vi "Sequencer Main.vi"() -> ()   [LabVIEW 2018] (continued)
                            n2810 = Replace Array Subset(array=w5930, new element=w5928, index=10) -> (w5931:errorcluster[])
                            n2811 = global write "Global Variable.vi" "Array Errors"(w5931) -> ()
                          }
                          n2812 = case shown="True" w5908 {
                            tunnel: [enum16{"Idle", "PASS", "FALSE"}."FALSE" ("Step Test Result") enum16{"Idle", "PASS", "FALSE"}."PASS" ("Step Test Result")] -> w5907
                            tunnel: ["FLASH FALSE" "FLASH OK"] -> w5904
                            frame False {
                              # "Step TEST Result"
                            }
                            frame True {
                              # "Step TEST Result"
                            }
                          }
                          n2813 = in-place {
                            in-place-border: w5906 -> [w5919]
                            in-place-border: w5905 -> [w5918]
                            in-place-border: w5904 -> [w5917]
                            n2814 = call "Log Add Msg.vi"("Result"=w5917, "Communication"=w5918, "Description"=w5919) -> ("Out Msg"=w5920:string)
                            n2815 = property on="LogMsg" class="Str"("Text.Scroll Position"=inf) -> ()  [unwired: 2 in, 2 out]
                            n2816 = invoke on="LogMsg" class="Str" method="Append String"("string"=w5920) -> ()  [unwired: 3 in, 4 out]
                          }
                        }
                        frame 1000 {
                          # "Power Supply OFF, Reset DIO"
                          # "Step TEST Result"
                          # "RESET POWER SUPPLY & RESET GPIO"
                          n2817 = Unbundle By Name(w5941) -> ("Step Description"=w5940:string)
                          n2818 = Concatenate Strings(w5940, "  " ("string"), "<END OF SEQUENCER>" ("string")) -> (w5942:string)
                          n2819 = local write "Message"(w5942) -> ()
                          n2820 = property on="Tab Control Msg" class="TabCtl (strict)"("Value"=T21."Msg" ("Tab Control Msg")) -> (error out=w5935:errorcluster)  [unwired: 2 in, 1 out]
                          n2821 = flat-sequence {
                            tunnel: w5935 -> [_]
                            tunnel: w5934 -> [w5960]
                            tunnel: w5933 -> [w5959]
                            frame #0 {
                              w5945 = FALSE ("Enable Output")
                              w5943 = 0.1 ("Current")
                              w5944 = 0.0 ("Voltage")
                              n2822 = global read "Global Variable.vi" "VISA Resource Name BK-9202"() -> (w5954:string)
                              n2823 = call "bk9201 Set.vi"("Enable Output"=w5945, "Current"=w5943, "Voltage"=w5944, "VISA resource name"=w5954) -> ("error out"=w5950:errorcluster)  [unwired: 7 in]
                              n2824 = local read "PowSupply - SET"() -> (w5947:T7)
                              n2825 = local read "Switch Relay Modules"() -> (w5949:T5)
                              n2826 = Bundle By Name(cluster=w5949, "Main Power Supplay ON/OFF"=w5945) -> (w5948:T5)
                              n2827 = global read "Global Variable.vi" "Array Errors"() -> (w5952:errorcluster[])
                              n2828 = Bundle By Name(cluster=w5947, "ON/OFF"=w5945, "Volt (V)"=w5944, "Current Limit (A)"=w5943) -> (w5946:T7)
                              n2829 = global write "Global Variable.vi" "PowSupply ON/OFF"(w5945) -> ()
                              n2830 = Replace Array Subset(array=w5952, new element=w5950, index=2) -> (w5953:errorcluster[])
                              n2831 = local write "Switch Relay Modules"(w5948) -> ()
                              n2832 = local write "PowSupply - SET"(w5946) -> ()
                              n2833 = global write "Global Variable.vi" "Array Errors"(w5953) -> ()
                            }
                            frame #1 {
                              n2834 = call <vilib>:"Acquire Semaphore.vi"("error in (no error)"=w5960, "semaphore"=w5959) -> ("error out"=w5958:errorcluster, "semaphore out"=w5956:T13)  [unwired: 3 in, 1 out]
                              n2835 = case shown="No Error" w5958 {
                                selector: w5958 -> [w5962 w5981]
                                tunnel: [w5962 w5981] -> w5955
                                tunnel: [w5961 w5980] -> w5957
                                tunnel: w5956 -> [w5961 w5980]
                                frame No Error {
                                n2836 = disable-structure shown="Disabled" {
                                frame Disabled {
                                n2837 = local read "Switch Relay Modules"() -> (w5970:T5)
                                n2838 = Number To Boolean Array(number=u16 0) -> (Boolean array=w5972:bool[])
                                n2839 = Bundle By Name(cluster=w5970, "SW 0"=w5972, "SW 1"=w5972, "SW 2"=w5972, "SW 3"=w5972, "SW 4"=w5972, "SW 5"=w5972, "SW 6"=w5972) -> (w5971:T5)
                                n2840 = local write "Switch Relay Modules"(w5971) -> ()
                                }
                                frame Enabled {
                                }
                                }
                                n2841 = global read "Global Variable.vi" "FTDI SPI Handle"() -> (w5965:u32)
                                n2842 = for {
                                N: 7 -> [_]
                                tunnel: w5965 -> [w5978]
                                tunnel: [w5979] -> w5968
                                i -> [w5973]
                                w5975 = u8 0  # nCS
                                w5974 = u16 0  # Channel Decimal
                                w5976 = FALSE  # Use Extra
                                n2843 = call "FTDI SPI GPIO Set.vi"("nCS"=w5975, "Mode"=T23."Set Decimal", "Use Extra"=w5976, "Channel Decimal"=w5974, "Addr"=w5973, "Handler In"=w5978) -> ("error out"=w5979:errorcluster)  [unwired: 2 in, 3 out]
                                }
                                n2844 = global read "Global Variable.vi" "Array Errors"() -> (w5966:errorcluster[])
                                n2845 = Replace Array Subset(array=w5966, new element=w5968, index=10) -> (w5967:errorcluster[])
                                n2846 = global write "Global Variable.vi" "Array Errors"(w5967) -> ()
                                }
                                frame Error {
                                }
                              }
                              n2847 = call <vilib>:"Release Semaphore.vi"("error in (no error)"=w5955, "semaphore"=w5957) -> ()  [unwired: 4 in, 2 out]
                            }
                            frame #2 {
                              w5982 = "!END OF TEST\nReset ALL"
                              n2848 = local write "Message"(w5982) -> ()
                              n2849 = property on="Msg Str" class="Str"("Value"=w5982) -> ()  [unwired: 2 in, 2 out]
                            }
                          }
                        }
                      }
                    }
                  }
                }
                frame #1 {
                  # "Step Result Msg"
                  # "Report"
                  # "Step TEST Result"
                  # "Run/Skip"
                  # "Step Type"
                  # "PASS/FALSE"
                  n2850 = Unbundle By Name(w5997) -> ("Run/Skip"=w5993:bool, "Step Type"=w5996:u16, "Report"=w5985:bool)
                  n2851 = flat-sequence {
                    tunnel: w5990 -> [w6002]
                    tunnel: w5983 -> [w6003]
                    tunnel: [w6005] -> w5995
                    tunnel: [w6004] -> w5994
                    tunnel: w5992 -> [w6000]
                    tunnel: [w6001] -> w5988
                    tunnel: w5995 -> [w6047]
                    tunnel: w5994 -> [w6048]
                    tunnel: w5983 -> [w6053]
                    tunnel: w5993 -> [w6049]
                    tunnel: w5991 -> [w6052]
                    tunnel: [w6051] -> w5984
                    tunnel: [w6050] -> w5989
                    tunnel: w5988 -> [w6050]
                    tunnel: w5983 -> [w6085]
                    tunnel: w5990 -> [w6084]
                    tunnel: w5989 -> [w6080]
                    tunnel: [w6079] -> w5986
                    tunnel: [w6114] -> w5987
                    tunnel: w5986 -> [w6114]
                    frame #0 {
                      # "BREACK ON FIRST Err"
                      n2852 = flat-sequence {
                        tunnel: w6000 -> [w6007]
                        tunnel: w6002 -> [w6008]
                        tunnel: w6003 -> [w6006]
                        tunnel: [w6008] -> w5999
                        tunnel: [w6007] -> w5998
                        tunnel: [w6019] -> w6005
                        tunnel: [w6018] -> w6004
                        tunnel: [w6016] -> w6001
                        tunnel: w5999 -> [w6017]
                        tunnel: w5998 -> [w6015]
                        frame #0 {
                          n2853 = case shown="\"FALSE\"" w6006 {
                            frame "Idle", Default {
                            }
                            frame "FALSE" {
                              n2854 = in-place {
                                in-place-border: [w6010] -> w6009
                                n2855 = global read "Global Variable.vi" "Retest Cnt"() -> (w6011:i16)
                                n2856 = Equal?(x=w6011, y=i16 0) -> (x = y?=w6010:bool)
                              }
                              n2857 = case shown="True" w6009 {
                                frame False {
                                }
                                frame True {
                                n2858 = global read "Global Variable.vi" "Gen Err Cnt"() -> (w6014:u16)
                                n2859 = Increment(x=w6014) -> (x+1=w6013:u16)
                                n2860 = global write "Global Variable.vi" "Gen Err Cnt"(w6013) -> ()
                                }
                              }
                            }
                          }
                        }
                        frame #1 {
                          # "GoTo  the last Sekuencer STEP (test Id=1000)"
                          n2861 = in-place {
                            in-place-border: [w6031] -> w6016
                            in-place-border: [w6029] -> w6019
                            in-place-border: [w6028] -> w6018
                            in-place-border: w6017 -> [w6027]
                            in-place-border: w6015 -> [w6026]
                            # "And"
                            # "Break On 3xFirst Err"
                            n2862 = global read "Global Variable.vi" "Gen Err Cnt"() -> (w6025:u16)
                            n2863 = Greater Or Equal?(x=w6025, y=u16 3) -> (x >= y?=w6021:bool)
                            n2864 = And(x=w6021, y="Break On First Err") -> (x .and. y?=w6022:bool)
                            n2865 = case shown="True" w6022 {
                              tunnel: [FALSE TRUE] -> w6023
                              frame False {
                              }
                              frame True {
                                n2866 = global write "Global Variable.vi" "Test Gen Status"(FALSE ("Test Gen Status")) -> ()
                              }
                            }
                            n2867 = And(x=w6023, y="Break On First Err") -> (x .and. y?=w6030:bool)
                            n2868 = case shown="True" w6030 {
                              tunnel: w6027 -> [_ w6045]
                              tunnel: w6026 -> [w6037 w6046]
                              tunnel: [w6037 w6042] -> w6031
                              tunnel: [FALSE TRUE] -> w6029
                              tunnel: [0 w6038] -> w6028
                              frame False {
                              }
                              frame True {
                                n2869 = global read "Sequencer Array.vi" "SEQUENCER Array"() -> (w6044:T16[])
                                n2870 = Flush Queue(queue=w6045, error in (no error)=w6046) -> (queue out=w6043:refnum<queue>, error out=w6041:errorcluster)  [unwired: 1 out]
                                n2871 = Array Size(array=w6044) -> (size(s)=w6040:i32)
                                n2872 = Decrement(x=w6040) -> (x-1=w6038:i32)
                                n2873 = property on="Test Sequencer" class="MCListbox (strict)"("Value"=w6038) -> ()  [unwired: 2 in, 2 out]
                                n2874 = Enqueue Element(queue=w6043, element=w6038, error in (no error)=w6041) -> (error out=w6042:errorcluster)  [unwired: 1 in, 2 out]
                              }
                            }
                          }
                        }
                      }
                    }
                    frame #1 {
                      # "Step TEST Result"
                      # "Run/Skip & Retest-ON"
                      # "Fill-Up (PASS/FALSE)Test Sequenser Table"
                      n2875 = case shown="True" w6047 {
                        tunnel: w6048 -> [_ w6056]
                        frame False {
                        }
                        frame True {
                          # "Break on first Err jump"
                          n2876 = Add(x=w6056, y=-5) -> (x+y=w6055:i32)
                          n2877 = Bundle By Name(cluster=T14 {"Row"=0, "Column"=0} ("Top Left Visible Cell"), "Row"=w6055, "Column"=u32 0) -> (w6059:T14)
                          n2878 = property on="Test Sequencer" class="MCListbox (strict)"("TopLeft"=w6059) -> ()  [unwired: 2 in, 2 out]
                        }
                      }
                      n2879 = case shown="True" w6049 {
                        tunnel: w6053 -> [_ w6068]
                        tunnel: [u32 16448250 w6064] -> w6051
                        tunnel: w6052 -> [_ w6061]
                        frame False {
                        }
                        frame True {
                          w6069 = 5 ("disabled index (col)")
                          # "Step Result Msg"
                          # "A-1"
                          n2880 = case shown="\"FALSE\"" w6068 {
                            tunnel: [u32 16448250 u32 46115 u32 16711680] -> w6064
                            tunnel: ["Idle" "PASS" "FALSE"] -> w6067
                            frame "Idle", Default {
                            }
                            frame "PASS" {
                            }
                            frame "FALSE" {
                            }
                          }
                          n2881 = global read "Global Variable.vi" "Current Step Nmb"() -> (w6063:u32)
                          n2882 = property on="Test Squencer Edit" class="MCListbox (strict)"() -> ("ItemNames"=w6065:string[][])  [unwired: 2 in, 2 out]
                          n2883 = Bundle By Name(cluster=T15 {"Row"=0, "Column"=0} ("Active Cell:Active Cell"), "Row"=w6063, "Column"=w6069) -> (w6070:T15)
                          n2884 = Replace Array Subset(array=w6065, new element #1=w6067, index (row) #1=w6063, index (col) #1=w6069, new element #2=w6061, index (row) #2=w6063, index (col) #2=3 ("disabled index (col)")) -> (w6066:string[][])
                          n2885 = property on="Test Squencer Edit" class="MCListbox (strict)"("ItemNames"=w6066, "ActiveCell"=w6070, "CellFontColor"=w6064) -> ()  [unwired: 2 in, 2 out]
                        }
                      }
                    }
                    frame #2 {
                      # "Step TEST Result"
                      n2886 = global read "Global Variable.vi" "Retest Cnt"() -> (w6078:i16)
                      n2887 = global read "Global Variable.vi" "Retest ON"() -> (w6082:bool)
                      n2888 = Greater Than 0?(x=w6078) -> (x > 0?=w6081:bool)
                      n2889 = And(x=w6082, y=w6081) -> (x .and. y?=w6083:bool)
                      n2890 = case shown="True" w6083 {
                        tunnel: w6085 -> [_ w6090]
                        tunnel: w6084 -> [_ w6089]
                        tunnel: w6080 -> [w6086 w6088]
                        tunnel: [w6086 w6087] -> w6079
                        frame False {
                        }
                        frame True {
                          n2891 = case shown="\"FALSE\"" w6090 {
                            tunnel: [w6091 w6094 w6112] -> w6087
                            tunnel: w6089 -> [_ w6093 _]
                            tunnel: w6088 -> [w6091 w6092 w6112]
                            frame "Idle", Default {
                            }
                            frame "FALSE" {
                              n2892 = in-place {
                                in-place-border: w6093 -> [w6102]
                                in-place-border: w6092 -> [w6101]
                                in-place-border: [w6096] -> w6094
                                # "RETEST"
                                n2893 = global read "Global Variable.vi" "Retest Step Nmb"() -> (w6095:u32)
                                n2894 = global read "Global Variable.vi" "Steps Nmb"() -> (w6098:u32)
                                n2895 = disable-structure shown="Disabled" {
                                disable-tunnel: w6095 -> [w6103 _]
                                frame Disabled {
                                n2896 = Bundle By Name(cluster=T14 {"Row"=0, "Column"=0} ("Top Left Visible Cell"), "Row"=w6103) -> (w6104:T14)
                                n2897 = property on="Test Sequencer" class="MCListbox (strict)"("TopLeft"=w6104) -> ()  [unwired: 2 in, 2 out]
                                }
                                frame Enabled {
                                }
                                }
                                n2898 = Flush Queue(queue=w6102, error in (no error)=w6101) -> (queue out=w6099:refnum<queue>, error out=w6100:errorcluster)  [unwired: 1 out]
                                n2899 = property on="Test Sequencer" class="MCListbox (strict)"("Value"=w6095) -> ()  [unwired: 2 in, 2 out]
                                n2900 = Subtract(x=w6098, y=w6095) -> (x-y=w6097:u32)
                                n2901 = for {
                                N: w6097 -> [_]
                                tunnel: w6100 -> [w6111]
                                tunnel: w6099 -> [w6110]
                                tunnel: w6095 -> [w6107]
                                tunnel: [w6106] -> w6096
                                i -> [w6109]
                                n2902 = Add(x=w6107, y=w6109) -> (x+y=w6108:u32)
                                n2903 = Enqueue Element(queue=w6110, element=w6108, error in (no error)=w6111) -> (error out=w6106:errorcluster)  [unwired: 1 in, 2 out]
                                }
                              }
                            }
                            frame "PASS" {
                              n2904 = global write "Global Variable.vi" "Retest Cnt"(i16 0 ("Retest Cnt")) -> ()
                            }
                          }
                        }
                      }
                    }
                    frame #3 {
                      n2905 = in-place {
                        n2906 = global read "Global Variable.vi" "Retest Nmb"() -> (w6115:i16)
                        n2907 = global read "Global Variable.vi" "Retest Cnt"() -> (w6117:i16)
                        n2908 = Subtract(x=w6115, y=w6117) -> (x-y=w6116:i16)
                        n2909 = Number To Decimal String(number=w6116) -> (decimal integer string=w6119:string)  [unwired: 1 in]
                        n2910 = Greater Than 0?(x=w6117) -> (x > 0?=w6120:bool)
                        "RETEST" <- w6120
                        n2911 = global write "Global Variable.vi" "Retest ON"(FALSE ("Retest Start")) -> ()
                        n2912 = case shown="False" w6120 {
                          tunnel: w6119 -> [w6121 w6122]
                          frame False {
                            n2913 = property on="RETEST" class="Bool (strict)"("BoolText.Text"=w6121) -> ()  [unwired: 2 in, 2 out]
                          }
                          frame True {
                            n2914 = property on="RETEST" class="Bool (strict)"("BoolText.Text"=w6122) -> ()  [unwired: 2 in, 2 out]
                          }
                        }
                      }
                    }
                  }
                }
                frame #2 {
                  # "Report"
                  # "Run / Skip"
                  # "A-1"
                  # "REPORT GENERATION"
                  n2915 = global read "Global Variable.vi" "Retest Cnt"() -> (w6127:i16)
                  n2916 = Equal To 0?(x=w6127) -> (x = 0?=w6125:bool)
                  n2917 = in-place {
                    in-place-border: w6129 -> [w6132]
                    # "Error Store"
                    n2918 = global read "Global Variable.vi" "Array Errors"() -> (w6134:errorcluster[])
                    n2919 = Replace Array Subset(array=w6134, new element=w6132, index=7) -> (w6135:errorcluster[])
                    n2920 = global write "Global Variable.vi" "Array Errors"(w6135) -> ()
                  }
                  n2921 = Compound Arithmetic op=AND(w6125, w6124, w6123) -> (w6126:bool)
                  n2922 = case shown="True" w6126 {
                    tunnel: w6131 -> [_ w6138]
                    tunnel: w6130 -> [_ w6137]
                    tunnel: w6128 -> [_ w6136]
                    frame False {
                    }
                    frame True {
                      n2923 = case shown="0" w6138 {
                        tunnel: w6137 -> [w6148 _ w6167]
                        tunnel: w6136 -> [w6144 _ _]
                        frame 100, Default {
                          # "All Steps (no Label)"
                          n2924 = case shown="\"FALSE\"" w6144 {
                            frame "Idle", Default {
                            }
                            frame "PASS" {
                            }
                            frame "FALSE" {
                              w6159 = u32 16746656
                              n2925 = Bundle(w6159, w6159) -> (w6160:cluster{u32, u32})  [unwired: 1 in]
                              n2926 = global write "Global Variable.vi" "Test Gen Status"(FALSE ("Test Gen Status")) -> ()
                              n2927 = Build Array(w6160) -> (w6161:cluster{u32, u32}[])
                              n2928 = property on="Gen Test Status" class="Bool (strict)"("Colors [4]"=w6161, "Value"=FALSE ("Gen Test Status")) -> ()  [unwired: 2 in, 2 out]
                            }
                          }
                          n2929 = global read "Global Variable.vi" "Current Step Nmb"() -> (w6155:u32)
                          n2930 = property on="Test Squencer Edit" class="MCListbox (strict)"() -> ("ItemNames"=w6156:string[][])  [unwired: 2 in, 2 out]
                          n2931 = global read "Global Variable.vi" "Report Step Nmb"() -> (w6146:u32)
                          n2932 = property on="Test Sequencer Run" class="MCListbox (strict)"() -> ("ItemNames"=w6154:string[][])  [unwired: 2 in, 2 out]
                          n2933 = Index Array(array=w6156, index (row)=w6155) -> (element=w6152:string[])  [unwired: 1 in]
                          n2934 = Increment(x=w6146) -> (x+1=w6145:u32)
                          n2935 = Number To Decimal String(number=w6146) -> (decimal integer string=w6143:string)  [unwired: 1 in]
                          n2936 = Replace Array Subset(array=w6152, new element=w6143, index=0) -> (w6142:string[])
                          n2937 = Array Subset(array=w6142, index=0, length=7) -> (w6139:string[])
                          n2938 = Bundle By Name(cluster=T15 {"Row"=0, "Column"=0} ("Active Cell:Active Cell"), "Row"=w6146, "Column"=5) -> (w6149:T15)
                          n2939 = Replace Array Subset(array=w6154, new element=w6139, index (row)=w6146) -> (w6153:string[][])  [unwired: 1 in]
                          n2940 = global write "Global Variable.vi" "Report Step Nmb"(w6145) -> ()
                          n2941 = property on="Test Sequencer Run" class="MCListbox (strict)"("ItemNames"=w6153, "ActiveCell"=w6149, "CellFontColor"=w6148, "Value"=w6146) -> ()  [unwired: 2 in, 2 out]
                        }
                        frame 1 {
                        }
                        frame 0 {
                          n2942 = global read "Global Variable.vi" "Current Step Nmb"() -> (w6178:u32)
                          n2943 = property on="Test Squencer Edit" class="MCListbox (strict)"() -> ("ItemNames"=w6179:string[][])  [unwired: 2 in, 2 out]
                          n2944 = global read "Global Variable.vi" "Report Step Nmb"() -> (w6169:u32)
                          n2945 = property on="Test Sequencer Run" class="MCListbox (strict)"() -> ("ItemNames"=w6177:string[][])  [unwired: 2 in, 2 out]
                          n2946 = Number To Decimal String(number=w6169) -> (decimal integer string=w6172:string)  [unwired: 1 in]
                          n2947 = for {
                            N: 7 -> [_]
                            tunnel: w6169 -> [w6182]
                            i -> [w6183]
                            n2948 = Bundle By Name(cluster=T15 {"Row"=0, "Column"=0} ("Active Cell:Active Cell"), "Row"=w6182, "Column"=w6183) -> (w6181:T15)
                            n2949 = property on="Test Sequencer Run" class="MCListbox (strict)"("ActiveCell"=w6181, "CellBG"=u32 16772930) -> ()  [unwired: 2 in, 2 out]
                          }
                          n2950 = Index Array(array=w6179, index (row)=w6178) -> (element=w6174:string[])  [unwired: 1 in]
                          n2951 = Increment(x=w6169) -> (x+1=w6175:u32)
                          n2952 = Replace Array Subset(array=w6174, new element=w6172, index=0) -> (w6164:string[])
                          n2953 = global write "Global Variable.vi" "Report Step Nmb"(w6175) -> ()
                          n2954 = Array Subset(array=w6164, index=0, length=7) -> (w6165:string[])
                          n2955 = Bundle By Name(cluster=T15 {"Row"=0, "Column"=0} ("Active Cell:Active Cell"), "Row"=w6169, "Column"=5) -> (w6170:T15)
                          n2956 = Replace Array Subset(array=w6177, new element=w6165, index (row)=w6169) -> (w6176:string[][])  [unwired: 1 in]
                          n2957 = property on="Test Sequencer Run" class="MCListbox (strict)"("ItemNames"=w6176, "Value"=w6169, "ActiveCell"=w6170, "CellFontColor"=w6167) -> ()  [unwired: 2 in, 2 out]
                        }
                      }
                    }
                  }
                }
                frame #3 {
                  # "Test Steps Manager"
                  n2958 = in-place {
                    w6195 = 20
                    w6198 = 20
                    n2959 = global read "Global Variable.vi" "Current Step Nmb"() -> (w6202:u32)
                    n2960 = global read "Global Variable.vi" "Report Step Nmb"() -> (w6191:u32)
                    n2961 = Quotient & Remainder(x=w6202, y=w6198) -> (floor(x/y)=w6199:u32)  [unwired: 1 out]
                    n2962 = Quotient & Remainder(x=w6191, y=w6195) -> (floor(x/y)=w6194:u32)  [unwired: 1 out]
                    n2963 = Multiply(x=w6199, y=w6198) -> (x*y=w6197:u32)
                    n2964 = Multiply(x=w6194, y=w6195) -> (x*y=w6196:u32)
                    n2965 = Bundle By Name(cluster=T14 {"Row"=0, "Column"=0} ("Top Left Visible Cell"), "Row"=w6197) -> (w6201:T14)
                    n2966 = Bundle By Name(cluster=T14 {"Row"=0, "Column"=0} ("Top Left Visible Cell"), "Row"=w6196) -> (w6192:T14)
                    n2967 = property on="Test Sequencer" class="MCListbox (strict)"("TopLeft"=w6201) -> ()  [unwired: 2 in, 2 out]
                    n2968 = property on="Test Sequencer Run" class="MCListbox (strict)"("TopLeft"=w6192) -> ()  [unwired: 2 in, 2 out]
                  }
                  n2969 = global read "Global Variable.vi" "Current Step Nmb"() -> (w6187:u32)
                  n2970 = global read "Global Variable.vi" "Steps Nmb"() -> (w6188:u32)
                  n2971 = in-place {
                    n2972 = local read "Tab Edit/Run"() -> (w6203:enum32{"Edit", "Run"})
                    n2973 = case shown="\"Edit\", Default" w6203 {
                      frame "Edit", Default {
                        n2974 = case shown="True" "Delay 1S" {
                          frame False {
                          }
                          frame True {
                            n2975 = Wait (ms)(milliseconds to wait=u32 1000) -> ()  [unwired: 1 out]
                          }
                        }
                      }
                      frame "Run" {
                      }
                    }
                  }
                  n2976 = in-place {
                    # "Prevent False durring run in RUN windows"
                    n2977 = local read "Tab Edit/Run"() -> (w6189:enum32{"Edit", "Run"})
                    n2978 = case shown="\"Run\"" w6189 {
                      frame "Edit", Default {
                      }
                      frame "Run" {
                        n2979 = Wait (ms)(milliseconds to wait=u32 100) -> ()  [unwired: 1 out]
                      }
                    }
                  }
                  n2980 = Decrement(x=w6188) -> (x-1=w6186:u32)
                  n2981 = Equal?(x=w6186, y=w6187) -> (x = y?=w6185:bool)
                  n2982 = case shown="True" w6185 {
                    frame False {
                      n2983 = global write "Global Variable.vi" "System Status"(T1."Run Sequencer" ("System Status")) -> ()
                    }
                    frame True {
                      n2984 = global write "Global Variable.vi" "System Status"(T1."STOP Sequencer" ("System Status")) -> ()
                    }
                  }
                  n2985 = in-place {
                    n2986 = Tick Count (ms)() -> (millisecond timer value=w6206:u32)
                    n2987 = global write "Global Variable.vi" "Test Stop Time"(w6206) -> ()
                  }
                }
              }
            }
          }
        }
        frame "STOP Sequencer" {
          n2988 = in-place {
            in-place-border: w6210 -> [w6212]
            in-place-border: w6209 -> [w6211]
            n2989 = flat-sequence {
              tunnel: w6212 -> [w6260]
              tunnel: w6211 -> [w6259]
              frame #0 {
                n2990 = global read "Global Variable.vi" "Test Gen Status"() -> (w6213:bool)
                n2991 = in-place {
                  # "Create Log File"
                  n2992 = call "Ini_LogFile.vi"() -> ("error out"=w6215:errorcluster, "logFile Path"=w6216:refnum<file>)  [unwired: 10 in]
                  n2993 = global write "Global Variable.vi" "logFile Path"(w6216) -> ()
                  n2994 = local read "LogMsg"() -> (w6220:string)
                  n2995 = Write to Text File(file (use dialog)=w6216, text=w6220, error in=w6215) -> (refnum out=w6218:refnum<file>, error out=w6219:errorcluster)  [unwired: 1 in, 1 out]
                  n2996 = Close File(refnum=w6218, error in=w6219) -> (error out=w6217:errorcluster)  [unwired: 1 out]
                  n2997 = call <userlib>:"Clear All Errors__ogtk.vi"("Error In"=w6217) -> ()  [unwired: 3 in, 1 out]
                }
                n2998 = case shown="True" w6213 {
                  frame False {
                    w6231 = u32 16711680
                    n2999 = Bundle(w6231, w6231) -> (w6232:cluster{u32, u32})  [unwired: 1 in]
                    n3000 = Build Array(w6232) -> (w6233:cluster{u32, u32}[])
                    n3001 = property on="Gen Test Status" class="Bool (strict)"("Colors [4]"=w6233, "Value"=FALSE ("Gen Test Status"), "Strings [4]"=string[] ["FALSE", "PASS", "", ""]) -> ()  [unwired: 2 in, 2 out]
                  }
                  frame True {
                    w6236 = u32 40735
                    n3002 = Bundle(w6236, w6236) -> (w6234:cluster{u32, u32})  [unwired: 1 in]
                    n3003 = Build Array(w6234) -> (w6235:cluster{u32, u32}[])
                    n3004 = property on="Gen Test Status" class="Bool (strict)"("Colors [4]"=w6235, "Value"=TRUE ("Gen Test Status"), "Strings [4]"=string[] ["FALSE", "PASS", "", ""]) -> ()  [unwired: 2 in, 2 out]
                  }
                }
                n3005 = case shown="True" FALSE {
                  frame False {
                  }
                  frame True {
                    n3006 = One Button Dialog(message="STOP Sequencer") -> ()  [unwired: 1 in, 1 out]
                  }
                }
                n3007 = in-place {
                  in-place-border: w6213 -> [w6221]
                  n3008 = local read "Cnt Total"() -> (w6222:i32)
                  n3009 = case shown="True" w6221 {
                    frame False {
                      n3010 = local read "Cnt False"() -> (w6225:i32)
                      n3011 = Increment(x=w6225) -> (x+1=w6224:i32)
                      n3012 = local write "Cnt False"(w6224) -> ()
                    }
                    frame True {
                      n3013 = local read "Cnt Pass"() -> (w6227:i32)
                      n3014 = Increment(x=w6227) -> (x+1=w6226:i32)
                      n3015 = local write "Cnt Pass"(w6226) -> ()
                    }
                  }
                  n3016 = Increment(x=w6222) -> (x+1=w6223:i32)
                  n3017 = local write "Cnt Total"(w6223) -> ()
                }
              }
              frame #1 {
                w6241 = FALSE ("Enable Output")
                w6239 = 0.1 ("Current")
                w6240 = 0.0 ("Voltage")
                n3018 = global read "Global Variable.vi" "VISA Resource Name BK-9202"() -> (w6250:string)
                n3019 = call "bk9201 Set.vi"("Enable Output"=w6241, "Current"=w6239, "Voltage"=w6240, "VISA resource name"=w6250) -> ("error out"=w6246:errorcluster)  [unwired: 7 in]
                n3020 = local read "PowSupply - SET"() -> (w6243:T7)
                n3021 = local read "Switch Relay Modules"() -> (w6245:T5)
                n3022 = Bundle By Name(cluster=w6245, "Main Power Supplay ON/OFF"=w6241) -> (w6244:T5)
                n3023 = global read "Global Variable.vi" "Array Errors"() -> (w6248:errorcluster[])
                n3024 = Bundle By Name(cluster=w6243, "ON/OFF"=w6241, "Volt (V)"=w6240, "Current Limit (A)"=w6239) -> (w6242:T7)
                n3025 = global write "Global Variable.vi" "PowSupply ON/OFF"(w6241) -> ()
                n3026 = Replace Array Subset(array=w6248, new element=w6246, index=2) -> (w6249:errorcluster[])
                n3027 = local write "Switch Relay Modules"(w6244) -> ()
                n3028 = local write "PowSupply - SET"(w6242) -> ()
                n3029 = global write "Global Variable.vi" "Array Errors"(w6249) -> ()
              }
              frame #2 {
                n3030 = global read "Global Variable.vi" "COM Port RFID"() -> (w6254:refnum<visa-resource-name>)
                n3031 = call "Stop Reading.vi"("error in (no error)"=errorcluster {"status"=FALSE, "code"=0, "source"=""}, "Baud Rate"=u32 38400, "COM Port"=w6254) -> ("error out"=w6251:errorcluster)  [unwired: 6 in, 2 out]
                n3032 = call <userlib>:"Clear All Errors__ogtk.vi"("Error In"=w6251) -> ()  [unwired: 3 in, 1 out]
              }
              frame #3 {
                n3033 = call <vilib>:"Acquire Semaphore.vi"("error in (no error)"=w6260, "semaphore"=w6259) -> ("error out"=w6258:errorcluster, "semaphore out"=w6257:T13)  [unwired: 3 in, 1 out]
                n3034 = case shown="No Error" w6258 {
                  selector: w6258 -> [w6272 w6319]
                  tunnel: w6257 -> [w6271 w6318]
                  tunnel: [w6272 w6319] -> w6256
                  tunnel: [w6271 w6318] -> w6255
                  frame No Error {
                    w6266 = u8 1  # nCS
                    w6267 = T20 0 items=["Addr-0"=0, "Addr-1"=4, "Addr-2"=2, "Addr-3"=6, "Addr-4"=1, "Addr-5"=5, "Addr-6"=3, "Addr-7"=7] ("Addr")
                    w6277 = T20 7 items=["Addr-0"=0, "Addr-1"=4, "Addr-2"=2, "Addr-3"=6, "Addr-4"=1, "Addr-5"=5, "Addr-6"=3, "Addr-7"=7] ("Addr")
                    # "FALSE"
                    # "PASS"
                    # "nCS"
                    n3035 = global read "Global Variable.vi" "FTDI SPI Handle"() -> (w6268:u32)
                    n3036 = for {
                      N: 4 -> [_]
                      tunnel: w6268 -> [w6296]
                      tunnel: [w6288] -> w6278
                      i -> [w6291]
                      w6293 = u8 0  # nCS
                      w6292 = u16 0  # Channel Decimal
                      w6294 = TRUE  # Use Extra
                      n3037 = call "FTDI SPI GPIO Set.vi"("nCS"=w6293, "Mode"=T23."Set Decimal", "Use Extra"=w6294, "Channel Decimal"=w6292, "Addr"=w6291, "Handler In"=w6296) -> ("error out"=w6288:errorcluster, "LATCH Reg"=w6289:u16)  [unwired: 2 in, 2 out]
                      n3038 = Number To Boolean Array(number=w6289) -> (Boolean array=w6290:bool[])
                      n3039 = case shown="0" w6291 {
                        tunnel: w6290 -> [_ w6297 w6300 w6303 w6306 w6309 w6312 w6315]
                        frame -1, Default {
                        }
                        frame 0 {
                          n3040 = local read "Switch Relay Modules"() -> (w6299:T5)
                          n3041 = Bundle By Name(cluster=w6299, "SW 0"=w6297) -> (w6298:T5)
                          n3042 = local write "Switch Relay Modules"(w6298) -> ()
                        }
                        frame 1 {
                          n3043 = local read "Switch Relay Modules"() -> (w6302:T5)
                          n3044 = Bundle By Name(cluster=w6302, "SW 1"=w6300) -> (w6301:T5)
                          n3045 = local write "Switch Relay Modules"(w6301) -> ()
                        }
                        frame 2 {
                          n3046 = local read "Switch Relay Modules"() -> (w6305:T5)
                          n3047 = Bundle By Name(cluster=w6305, "SW 2"=w6303) -> (w6304:T5)
                          n3048 = local write "Switch Relay Modules"(w6304) -> ()
                        }
                        frame 3 {
                          n3049 = local read "Switch Relay Modules"() -> (w6308:T5)
                          n3050 = Bundle By Name(cluster=w6308, "SW 3"=w6306) -> (w6307:T5)
                          n3051 = local write "Switch Relay Modules"(w6307) -> ()
                        }
                        frame 4 {
                          n3052 = local read "Switch Relay Modules"() -> (w6311:T5)
                          n3053 = Bundle By Name(cluster=w6311, "SW 4"=w6309) -> (w6310:T5)
                          n3054 = local write "Switch Relay Modules"(w6310) -> ()
                        }
                        frame 5 {
                          n3055 = local read "Switch Relay Modules"() -> (w6314:T5)
                          n3056 = Bundle By Name(cluster=w6314, "SW 5"=w6312) -> (w6313:T5)
                          n3057 = local write "Switch Relay Modules"(w6313) -> ()
                        }
                        frame 6 {
                          n3058 = local read "Switch Relay Modules"() -> (w6317:T5)
                          n3059 = Bundle By Name(cluster=w6317, "SW 6"=w6315) -> (w6316:T5)
                          n3060 = local write "Switch Relay Modules"(w6316) -> ()
                        }
                      }
                    }
                    n3061 = local read "Gen Test Status"() -> (w6263:bool)
                    n3062 = global read "Global Variable.vi" "FTDI SPI Handle"() -> (w6283:u32)
                    n3063 = Select(t=1, s=w6263, f=2) -> (s? t:f=w6264:i32)
                    n3064 = call "FTDI SPI GPIO Set.vi"("nCS"=u8 2, "Mode"=T24."Set Decimal", "Use Extra"=TRUE, "Channel Decimal"=w6264, "Addr"=w6277, "Handler In"=w6283) -> ("error out"=w6279:errorcluster, "LATCH Reg"=w6276:u16)  [unwired: 2 in, 2 out]
                    n3065 = local read "Switch Relay Modules"() -> (w6274:T5)
                    n3066 = Number To Boolean Array(number=w6276) -> (Boolean array=w6275:bool[])
                    n3067 = Bundle By Name(cluster=w6274, "SW 7"=w6275) -> (w6273:T5)
                    n3068 = global read "Global Variable.vi" "Array Errors"() -> (w6286:errorcluster[])
                    n3069 = Merge Errors(w6278, w6279) -> (w6280:errorcluster)
                    n3070 = local write "Switch Relay Modules"(w6273) -> ()
                    n3071 = Replace Array Subset(array=w6286, new element=w6280, index=10) -> (w6287:errorcluster[])
                    n3072 = call "FTDI SPI GPIO Set.vi"("nCS"=w6266, "Use Extra"=TRUE, "Channel Decimal"=u16 0, "Addr"=w6267, "Handler In"=w6268) -> ()  [unwired: 3 in, 4 out]
                    n3073 = global write "Global Variable.vi" "Array Errors"(w6287) -> ()
                  }
                  frame Error {
                  }
                }
                n3074 = call <vilib>:"Release Semaphore.vi"("error in (no error)"=w6256, "semaphore"=w6255) -> ()  [unwired: 4 in, 2 out]
              }
              frame #4 {
                n3075 = local read "Restart Cnt"() -> (w6321:u16)
                n3076 = local read "Auto\nRestart"() -> (w6322:u16)
                n3077 = Less?(x=w6321, y=w6322) -> (x < y?=w6323:bool)
                n3078 = case shown="True" w6323 {
                  frame False {
                    n3079 = local read "Report Auto"() -> (w6327:bool)
                    n3080 = case shown="True" w6327 {
                      frame False {
                        n3081 = global write "Global Variable.vi" "System Status"(T1."Idle" ("System Status")) -> ()
                      }
                      frame True {
                        n3082 = global read "Global Variable.vi" "Retest Nmb"() -> (w6329:i16)
                        n3083 = case shown="0, Default" w6329 {
                          frame 0, Default {
                            n3084 = property on="Tab Control Main" class="TabCtl (strict)"("Value"=T2."Report" ("Tab Control Main")) -> ()  [unwired: 2 in, 2 out]
                            n3085 = global write "Global Variable.vi" "System Status"(T1."Report Generation" ("System Status")) -> ()
                          }
                          frame 1 {
                            n3086 = global write "Global Variable.vi" "Test Gen Status"(FALSE ("Test Gen Status")) -> ()
                            n3087 = global write "Global Variable.vi" "System Status"(T1."Idle" ("System Status")) -> ()
                          }
                        }
                      }
                    }
                    n3088 = local write "Auto\nRestart"(1) -> ()
                    n3089 = local write "Message"(">>>STOP SEQUENSER <<<") -> ()
                    n3090 = property on="Run Test" class="Bool"("DisabledEnum"=T18."Enabled" ("Disabled")) -> ()  [unwired: 2 in, 2 out]
                  }
                  frame True {
                    n3091 = local write "Auto\nReStart"(TRUE ("Auto\nReStart")) -> ()
                    n3092 = global write "Global Variable.vi" "Reset BARCODE"(TRUE ("Reset BARCODE")) -> ()
                    n3093 = local read "Report Auto"() -> (w6335:bool)
                    n3094 = case shown="False" w6335 {
                      frame False {
                        # "Idle"
                        n3095 = global write "Global Variable.vi" "System Status"(T1."Idle" ("System Status")) -> ()
                        n3096 = property on="Tab Control Main" class="TabCtl (strict)"("Value"=T2."TEST Board" ("Tab Control Main")) -> ()  [unwired: 2 in, 2 out]
                      }
                      frame True {
                        n3097 = global write "Global Variable.vi" "System Status"(T1."Report Generation" ("System Status")) -> ()
                        n3098 = property on="Tab Control Main" class="TabCtl (strict)"("Value"=T2."Report" ("Tab Control Main")) -> ()  [unwired: 2 in, 2 out]
                      }
                    }
                    n3099 = local write "Message"(">>> RESTART TEST Sequencer <<<") -> ()
                  }
                }
                n3100 = property on="Msg Str" class="Str"("Value"="STOP SEQUENSER\nReset ALL") -> ()  [unwired: 2 in, 2 out]
              }
            }
          }
        }
        frame "Report Generation" {
          n3101 = flat-sequence {
            tunnel: [w6356] -> w6349
            tunnel: [w6355] -> w6348
            tunnel: [w6352] -> w6347
            tunnel: [w6390] -> w6351
            tunnel: [w6389] -> w6350
            tunnel: w6349 -> [w6389]
            tunnel: w6348 -> [w6388]
            tunnel: w6347 -> [w6386]
            tunnel: w6351 -> [w6400]
            tunnel: [w6399] -> w6346
            tunnel: w6350 -> [w6399]
            tunnel: w6346 -> [w6407]
            tunnel: [w6408] -> w6345
            tunnel: [w6407] -> w6344
            tunnel: [w6405] -> w6343
            tunnel: [w6406] -> w6342
            tunnel: w6345 -> [w6447]
            tunnel: w6344 -> [w6446]
            tunnel: w6343 -> [w6444]
            tunnel: w6342 -> [w6445]
            frame #0 {
              w6353 = "<p>&nbsp;</p>" ("string")
              w6379 = u16 2 items=["Default", "US", "Metric"] ("measurement system (default)")
              # "table {\n  font-family: arial, sans-serif;\n  border-collapse: collapse;\n  width: 70%;\n}"
              # "Hardware Revision"
              n3102 = property on="Test Sequencer Run" class="MCListbox (strict)"() -> ("ColHdrString"=w6385:string[], "ItemNames"=w6381:string[][])  [unwired: 2 in, 2 out]
              n3103 = local read "Test Time"() -> (w6361:string)
              n3104 = call <vilib>:"New Report.vi"("report type"=T31."HTML") -> ("report out"=w6375:refnum<class "NI_report.lvclass">, "error out"=w6378:errorcluster)  [unwired: 5 in, 8 out]
              n3105 = local read "Customer"() -> (w6372:string)
              n3106 = local read "Under Test BOARD"() -> (w6371:string)
              n3107 = local read "Barcode"() -> (w6368:string)
              n3108 = property on="Operator" class="Ring (strict)"() -> ("RingText.Text"=w6367:string)  [unwired: 2 in, 2 out]
              n3109 = local read "Config"() -> (w6370:string)
              n3110 = global read "Global Variable.vi" "Report Step Nmb"() -> (w6358:u32)
              n3111 = call-dynamic "Set Report Margins.vi"("report in"=w6375, "margins (1.00)"=T32 {"top"=10.0, "left"=10.0, "right"=10.0, "bottom"=10.0}, "measurement system (default)"=w6379, "error in (no error)"=w6378) -> ("report out"=w6376:refnum<class "NI_report.lvclass">, "error out"=w6377:errorcluster)  [unwired: 9 in, 1 out]
              n3112 = local read "Gen Test Status"() -> (w6366:bool)
              n3113 = Array Subset(array=w6385, index=0, length=7) -> (w6382:string[])
              n3114 = Concatenate Strings("Measurement Results" ("Table Header"), "    (", "TestTime -" ("Table Header"), w6361, ")") -> (w6363:string)
              n3115 = Increment(x=w6358) -> (x+1=w6357:u32)
              n3116 = Build Array (concatenate)(w6382, w6381) -> (w6380:string[][])
              n3117 = call "html Header.vi"("Test Result"=w6366, "Test Operator"=w6367, "Company"=w6372, "Serial Numbe (SN)"=w6368, "Hardware Revision"="v1.1", "Product Info"=w6370, "Product Name"=w6371) -> ("html string"=w6354:string)  [unwired: 4 in]
              n3118 = call "html Table.vi"("Rows cnt"=w6357, "Table Header"=w6363, "In String Table"=w6380) -> ("html string out"=w6365:string)  [unwired: 8 in]
              n3119 = Concatenate Strings(w6354, w6353, w6365, w6353) -> (w6356:string)
              n3120 = call-dynamic "Append User Formatted HTML to Report.vi"("report in"=w6376, "HTML text"=w6356, "error in (no error)"=w6377) -> ("report out"=w6352:refnum<class "NI_report.lvclass">, "error out"=w6355:errorcluster)  [unwired: 11 out]
            }
            frame #1 {
              n3121 = in-place {
                in-place-border: w6386 -> [w6396]
                in-place-border: [w6395] -> w6390
                # "Local Temp File"
                n3122 = call <vilib>:"Application Directory.vi"() -> ("Application Directory"=w6398:path)
                n3123 = Build Path(base path=w6398, name or relative path="report.html") -> (appended path=w6395:path)
                n3124 = call-dynamic "Save Report to File.vi"("report in"=w6396, "report file path"=w6395) -> ()  [unwired: 12 in, 2 out]
                n3125 = Wait (ms)(milliseconds to wait=u32 250) -> ()  [unwired: 1 out]
              }
              n3126 = case shown="True" "Open in Default IE" {
                tunnel: w6388 -> [_ w6393]
                tunnel: w6386 -> [_ w6392]
                frame False {
                  n3127 = Wait (ms)(milliseconds to wait=u32 2000) -> ()  [unwired: 1 out]
                }
                frame True {
                  # "Open HTML Report in Browser VI"
                  n3128 = call-poly <vilib>:"Open HTML Report in Browser.vi"("report in"=w6392, "error in (no error)"=w6393) -> ()  [unwired: 14 out]
                }
              }
            }
            frame #2 {
              n3129 = Path To String(path=w6400) -> (string=w6403:string)
              n3130 = invoke class="IWebBrowser2" method="Navigate"(reference="WebBrowser", "URL"=w6403) -> (error out=w6401:errorcluster)  [unwired: 6 in, 7 out]
              n3131 = call <userlib>:"Clear All Errors__ogtk.vi"("Error In"=w6401) -> ()  [unwired: 3 in, 1 out]
            }
            frame #3 {
              # "Create BARCODE / Number FOLDER"
              n3132 = global read "Global Variable.vi" "DB Dir Path"() -> (w6404:path)
              n3133 = in-place {
                in-place-border: [w6426] -> w6406
                in-place-border: [w6413] -> w6405
                in-place-border: w6404 -> [w6411]
                # "Sub Dir?"
                # "FALSE Sub Dir?"
                n3134 = Get Date/Time String() -> (date string=w6421:string)  [unwired: 3 in, 1 out]
                n3135 = while {
                  shift-right: [w6437] -> w6422
                  shift-left: w6421 -> [w6440]
                  stop <- w6435 stop-if-true
                  # "Replase character / to _"
                  n3136 = call <vilib>:"Search and Replace Pattern.vi"("string"=w6440, "regular expression (\"\")"="/" ("substring (\"\")"), "replace string (\"\")"="_" ("replace string (\"\")")) -> ("result string"=w6437:string, "offset past match"=w6436:i32)  [unwired: 2 in]
                  n3137 = Less Than 0?(x=w6436) -> (x < 0?=w6435:bool)
                }
                n3138 = local read "Config"() -> (w6415:string)
                n3139 = Build Path(base path=w6411, name or relative path=w6422) -> (appended path=w6416:path)
                n3140 = Build Path(base path=w6416, name or relative path=w6415) -> (appended path=w6414:path)
                n3141 = call <vilib>:"Check if File or Folder Exists.vi"("path"=w6414) -> ("file or folder exists?"=w6420:bool, "dup path"=w6425:path)  [unwired: 8 in, 1 out]
                n3142 = Not(x=w6420) -> (.not. x?=w6424:bool)
                n3143 = case shown="True" w6424 {
                  tunnel: w6425 -> [w6431 w6434]
                  tunnel: [w6431 w6432] -> w6413
                  frame False {
                  }
                  frame True {
                    # "Time/Date Sub Dir"
                    n3144 = Create Folder(path (use dialog)=w6434) -> (created path=w6432:path, error out=w6433:errorcluster)  [unwired: 2 in, 1 out]
                    n3145 = call <userlib>:"Clear All Errors__ogtk.vi"("Error In"=w6433) -> ()  [unwired: 3 in, 1 out]
                  }
                }
                n3146 = Build Path(base path=w6413, name or relative path="FALSE") -> (appended path=w6418:path)
                n3147 = call <vilib>:"Check if File or Folder Exists.vi"("path"=w6418) -> ("file or folder exists?"=w6417:bool, "dup path"=w6412:path)  [unwired: 8 in, 1 out]
                n3148 = Not(x=w6417) -> (.not. x?=w6423:bool)
                n3149 = case shown="True" w6423 {
                  tunnel: w6412 -> [w6427 w6430]
                  tunnel: [w6427 w6428] -> w6426
                  frame False {
                  }
                  frame True {
                    # "FALSE Sub Dir"
                    n3150 = Create Folder(path (use dialog)=w6430) -> (created path=w6428:path, error out=w6429:errorcluster)  [unwired: 2 in, 1 out]
                    n3151 = call <userlib>:"Clear All Errors__ogtk.vi"("Error In"=w6429) -> ()  [unwired: 3 in, 1 out]
                  }
                }
              }
              n3152 = local read "Barcode"() -> (w6410:string)
              n3153 = in-place {
                in-place-border: w6410 -> [w6443]
                in-place-border: [w6441] -> w6408
                # "Length of Barcode > ?"
                n3154 = String Length(string=w6443) -> (length=w6442:i32)
                n3155 = Greater Than 0?(x=w6442) -> (x > 0?=w6441:bool)
              }
              n3156 = Wait (ms)(milliseconds to wait=u32 3000) -> ()  [unwired: 1 out]
            }
            frame #4 {
              # "Date"
              n3157 = case shown="True" w6447 {
                tunnel: w6446 -> [_ w6459]
                tunnel: w6445 -> [_ w6449]
                tunnel: w6444 -> [_ w6448]
                frame False {
                }
                frame True {
                  n3158 = call <vilib>:"New Report.vi"("report type"=T31."HTML") -> ("report out"=w6461:refnum<class "NI_report.lvclass">, "error out"=w6462:errorcluster)  [unwired: 5 in, 8 out]
                  n3159 = local read "Barcode"() -> (w6458:string)
                  n3160 = local read "Gen Test Status"() -> (w6454:bool)
                  n3161 = call-dynamic "Set Report Margins.vi"("report in"=w6461, "error in (no error)"=w6462) -> ("report out"=w6464:refnum<class "NI_report.lvclass">, "error out"=w6463:errorcluster)  [unwired: 11 in, 1 out]
                  n3162 = call-dynamic "Append User Formatted HTML to Report.vi"("report in"=w6464, "HTML text"=w6459, "error in (no error)"=w6463) -> ("report out"=w6451:refnum<class "NI_report.lvclass">, "error out"=w6460:errorcluster)  [unwired: 11 out]
                  n3163 = Concatenate Strings(w6458, ".html" ("string")) -> (w6452:string)
                  n3164 = Not(x=w6454) -> (.not. x?=w6453:bool)
                  n3165 = Build Path(base path=w6448, name or relative path=w6452) -> (appended path=w6455:path)
                  n3166 = call-dynamic "Save Report to File.vi"("report in"=w6451, "report file path"=w6455, "prompt to replace? (F)"=FALSE, "error in (no error)"=w6460) -> ("error out"=w6450:errorcluster)  [unwired: 10 in, 1 out]
                  n3167 = case shown="True" w6453 {
                    tunnel: w6449 -> [_ w6471]
                    tunnel: w6451 -> [_ w6469]
                    tunnel: w6452 -> [_ w6468]
                    frame False {
                    }
                    frame True {
                      n3168 = Build Path(base path=w6471, name or relative path=w6468) -> (appended path=w6470:path)
                      n3169 = call-dynamic "Save Report to File.vi"("report in"=w6469, "report file path"=w6470, "prompt to replace? (F)"=FALSE) -> ("error out"=w6466:errorcluster)  [unwired: 11 in, 1 out]
                      n3170 = call <userlib>:"Clear All Errors__ogtk.vi"("Error In"=w6466) -> ()  [unwired: 3 in, 1 out]
